vi "Enter Authentication Code.vi"(8 "error in (no error)":errorcluster) -> (0 "error out":errorcluster, 2 "Cencel":bool, 3 "Authentication Code":string)   [LabVIEW 2015, in "Telegram Library.lvlib"]
doc: "Created IvanLis by LabVIEW Portal\nProfile: http://labviewportal.org/memberlist.php?mode=viewprofile&u=987\neMail: IvanLisanov@gMail.com\nTelegram: https://t.me/IvanLis"
uses:
  Telegram Library.lvlib
panel:
  in  "Cancel Button":bool
  in  "OK Button":bool
  in  "Enter Authentication Code":string
  # "Enter Authentication Code"
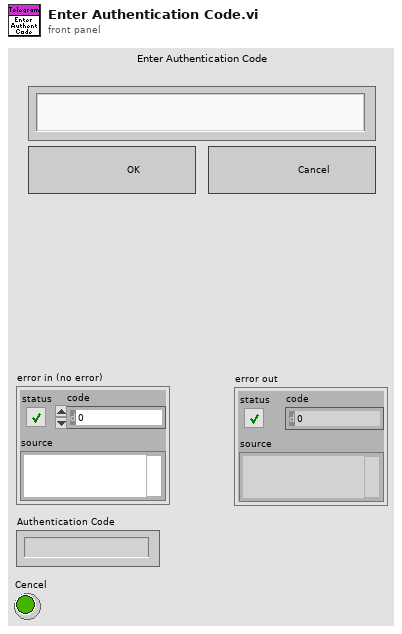
[diagram p1: front panel]
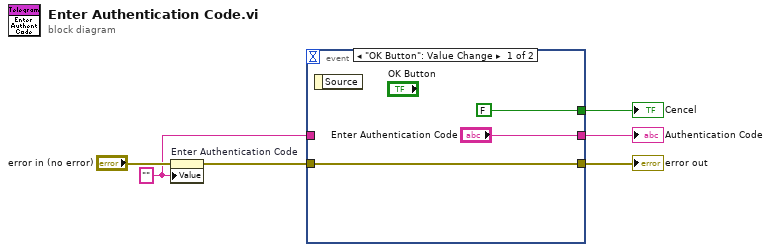
[diagram p0: block diagram]
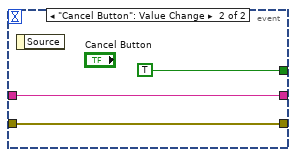
[diagram p2: hidden frame]
diagram:
  w4 = "" ("Enter Authentication Code")
  n1 = property on="Enter Authentication Code" class="Str"(error in="error in (no error)", "Value"=w4) -> (error out=w5:errorcluster)  [unwired: 1 in, 1 out]
  n2 = event shown="[0] \"OK Button\": Value Change" {
    selector: _ -> [_ _]
    dyn-events: _ -> [_ _]
    timeout: _ -> [_ _]
    tunnel: w5 -> [w9 w12]
    tunnel: [w9 w12] -> w1
    tunnel: ["Enter Authentication Code" w11] -> w2
    tunnel: w4 -> [_ w11]
    tunnel: [FALSE TRUE] -> w3
    event "OK Button": Value Change {
      n3 = event-data() -> ()  [unwired: 1 in, 1 out]
    }
    event "Cancel Button": Value Change {
      n4 = event-data() -> ()  [unwired: 1 in, 1 out]
    }
  }
  "error out" <- w1
  "Authentication Code" <- w2
  "Cencel" <- w3
